vi "Open.vi"(8 "error in (no error)":errorcluster caption="entrée d'erreur (pas d'erreur)", 11 "Class Spectrum_Analyser RS306B en entrée":refnum<class "Class Spectrum_Analyser RS306B.lvclass">) -> (0 "error out":errorcluster caption="sortie d'erreur", 3 "Class Spectrum_Analyser RS306B en sortie":refnum<class "Class Spectrum_Analyser RS306B.lvclass">)   [LabVIEW 2020, in "Library Instrument & Equipement.lvlib" / "Library Spectrum Analyser.lvlib" / "Class Spectrum_Analyser RS306B.lvclass"]
uses:
  Class Spectrum_Analyser RS306B.lvclass
  C:/Users/ngarcin/OneDrive - Altyor/Standard TB/Class/Spectrum Analyser/Class Spectrum Analyser (Default)/Class Spectrum Analyser (Default).lvclass
  Class Spectrum_Analyser RS306B.lvclass/Class Spectrum_Analyser RS306B.ctl
  Library Spectrum Analyser.lvlib
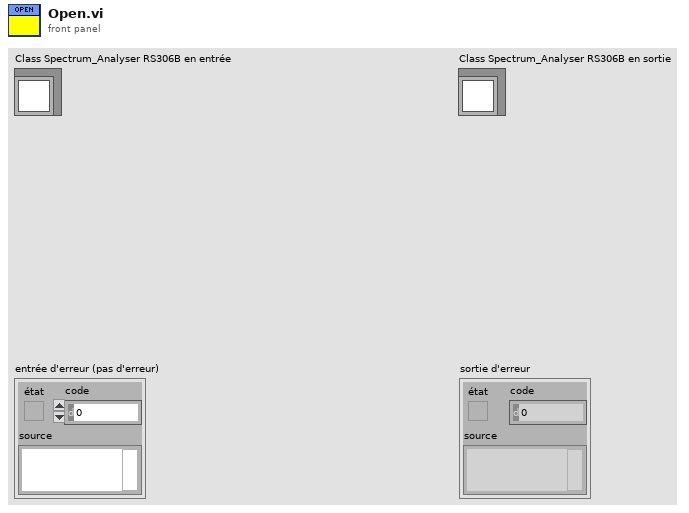
[diagram p1: front panel]
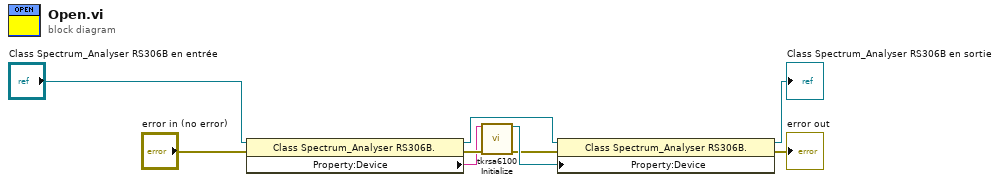
[diagram p0: block diagram]
diagram:
  n1 = property class="Class Spectrum_Analyser RS306B."(reference="Class Spectrum_Analyser RS306B en entrée", error in="error in (no error)") -> (reference out=w6:refnum<class "Class Spectrum_Analyser RS306B.lvclass">, error out=w5:errorcluster, "Property:Device"=w1:string)
  n2 = call "tkrsa6100 Initialize.vi"("VISA Resource Name"=w1, "error in (no error)"=w5) -> ("dup VISA Resource Name"=w8:refnum<visa-resource-name>, "error out"=w3:errorcluster)  [unwired: 9 in, 3 out]
  n3 = property class="Class Spectrum_Analyser RS306B."(reference=w6, error in=w3, "Property:Device"=w8) -> (reference out=→"Class Spectrum_Analyser RS306B en sortie":refnum<class "Class Spectrum_Analyser RS306B.lvclass">, error out=→"error out":errorcluster)
